vi "ide_comandos.vi"() -> ()   [LabVIEW 2011]
uses:
  <vilib>/addons/System Identification/Model Conversion.llb/SI Convert to Transfer Function Model of CDT.vi
  <vilib>/addons/Control Design/_Utility/Model Viewer.llb/Model Viewer SubVI/cd_Draw Transfer Function Equation (TF).vi
  <vilib>/addons/Control Design/_Time Response Analysis/Time Response.llb/Time Response subVI/cd_Step Response (Transfer Function).vi
  <vilib>/addons/System Identification/NI_SysID.lvlib
  <vilib>/addons/Control Design/_Time Response Analysis/NI_CD_Time Response.lvlib
  <vilib>/addons/Control Design/_Utility/NI_CD_Model Viewer.lvlib
panel:
  out "MODELO ARX TIEMPO DISCRETO":picture
  out "FUNCION DE TRANSF. TIEMPO CONT.":picture
  in  "model type":u16(ring)=1 items=["State-Space", "Transfer Function", "Zero-Pole-Gain"]
  out "RESPUESTA AL ESCALON":cluster{"time":dbl[], dbl[]}[](graph)=[{"time"=[0.0, 0.020293175540355358, 0.040586351080710716, 0.06087952662106608, 0.08117270216142143, 0.10146587770177679, 0.12175905324213215, 0.1420522287824875, 0.16234540432284286, 0.18263857986319823, 0.20293175540355357, 0.22322493094390894, 0.2435181064842643, 0.2638112820246197, 0.284104457564975, 0.30439763310533036, 0.3246908086456857, 0.3449839841860411, 0.36527715972639646, 0.3855703352667518, 0.40586351080710714, 0.4261566863474625, 0.4464498618878179, 0.46674303742817325, 0.4870362129685286, 0.507329388508884, 0.5276225640492394, 0.5479157395895946, 0.56820891512995, 0.5885020906703053, 0.6087952662106607, 0.6290884417510161, 0.6493816172913714, 0.6696747928317268, 0.6899679683720822, 0.7102611439124376, 0.7305543194527929, 0.7508474949931483, 0.7711406705335035, 0.7914338460738589, 0.8117270216142143], [0.0, 0.18042870525480673, 0.32815123498496285, 0.44909621299752056, 0.548117585926744, 0.6291894291559041, 0.6955654404163361, 0.7499095221019031, 0.7944026930256598, 0.8308306203628951, 0.8606552847447804, 0.8850736546744598, 0.9050657250759233, 0.9214338479313019, 0.9348349334831595, 0.9458068143490943, 0.9547898306331434, 0.9621445023202948, 0.9681659982093576, 0.9730959820732661, 0.9771323114748264, 0.9804369784854365, 0.9831426109957054, 0.9853577955383902, 0.9871714352472293, 0.9886563178518591, 0.9898720369049804, 0.9908673834808734, 0.9916823043325279, 0.9923495050951021, 0.9928957628778988, 0.9933430009237824, 0.993709168465894, 0.9940089610933998, 0.9942544105370846, 0.9944553675449554, 0.9946198972273457, 0.9947546027381128, 0.9948648902823868, 0.9949551860865656, 0.9950291140383205]}]
  in  "Filename":path=path "B:/UNI/Control Digital/2013-II/Laboratorios en el MT/7/circuito_rc.sim"
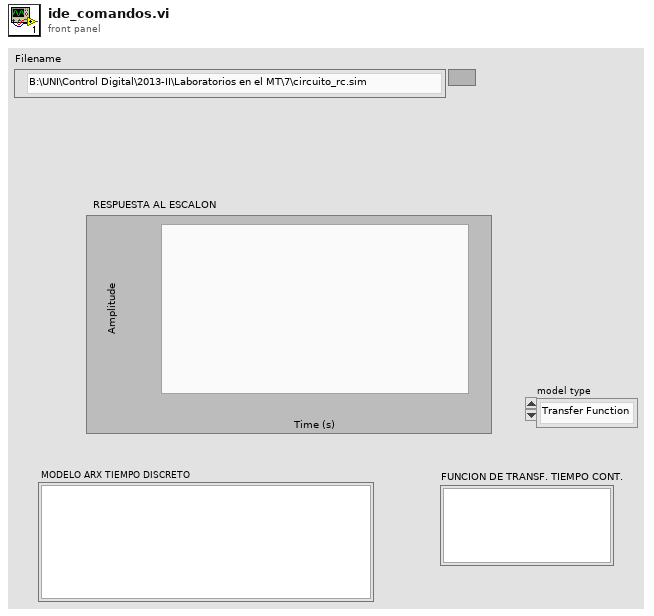
[diagram p1: front panel]
types:
  T1 = typedef "NI_SysID.lvlib/si_generic model.ctl" = cluster{"attributes":cluster{"version":string, "model type":T2, "input names":string[], "output names":string[], "notes":string}, "coefficients":cluster{"A ":dbl[][][], "B":dbl[][][], "F":dbl[][][], "C":dbl[][][], "D":dbl[][][]}, "std deviations":cluster{"A ":dbl[][][], "B":dbl[][][], "F":dbl[][][], "C":dbl[][][], "D":dbl[][][]}, "coefficients covariance":dbl[][][], "noise variance":dbl[][], "fs":dbl, "system info":cluster{"number of inputs":i32, "number of outputs":i32, "A order":i32[][], "B order":i32[][], "F order":i32[][], "C order":i32[][], "D order":i32[][], "Delays":i32[][]}, "kalman gain":dbl[][], "initial state":dbl[], "trans func":cluster{"betas":dbl[], "alphas":dbl[]}[][], "zeros-poles":cluster{"zeros":cdb[], "poles":cdb[], "gain":dbl}[][], "std of trans func":cluster{"betas":dbl[], "alphas":dbl[]}[][], "std of zeros-poles":cluster{"zeros":cdb[], "poles":cdb[], "gain":dbl}[][], "trans func (noise)":cluster{"betas":dbl[], "alphas":dbl[]}[][], "std of trans func (noise)":cluster{"betas":dbl[], "alphas":dbl[]}[][], "zeros-poles (noise)":cluster{"zeros":cdb[], "poles":cdb[], "gain":dbl}[][], "std of zeros-poles (noise)":cluster{"zeros":cdb[], "poles":cdb[], "gain":dbl}[][], "Symbolic State Space Model":cluster{"Symbolic A":string[][], "Symbolic B":string[][], "Symbolic C":string[][], "Symbolic D":string[][], "Symbolic K":string[][], "Symbolic Initial State":string[]}, "delay":dbl[][], "variables":T3, "grey trans func spec":cluster{"orders of TF model":cluster{" num order":i32, "den order":i32}, "# of zeros/poles at origin":cluster{"zeros/poles":u16, "number ":i32}, "delay initial?":bool, "gain initial?":bool}}
  T2 = typedef "NI_SysID.lvlib/SI Model Type.ctl" = u16
  T3 = typedef "NI_SysID.lvlib/si_variables.ctl" = cluster{"name":string, "initial guess":dbl, "upper limit":dbl, "lower limit":dbl, "value":dbl}[]
  T4 = typedef "NI_LinSys_Model Typedefs.lvlib/CD Transfer Function Model (MIMO).ctl" = cluster{"properties":T5, "transfer function(s)":T6[][]}
  T5 = typedef "NI_LinSys_Model Typedefs.lvlib/CD General Elements.ctl" = cluster{"Model name":string, "Input names":string[], "Output names":string[], "Input Delays":dbl[], "Output Delays":dbl[], "Sampling Time":dbl, "Notes":string}
  T6 = typedef "NI_LinSys_Model Typedefs.lvlib/CD Transfer Function Model (SISO).ctl" = cluster{"Numerator":dbl[], "Denominator":dbl[], "delay":dbl}
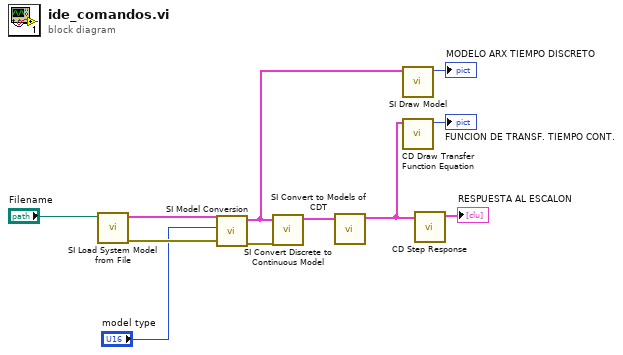
[diagram p0: block diagram]
diagram:
  n1 = call <vilib>:"SI Load System Model from File.vi"("file path"="Filename") -> ("error out"=w9:errorcluster, "system model"=w8:T1)  [unwired: 7 in, 2 out]
  n2 = call <vilib>:"SI Model Conversion.vi"("error in (no error)"=w9, "model type"="model type", "system model in"=w8) -> ("error out"=w11:errorcluster, "system model out"=w7:T1)  [unwired: 7 in]
  n3 = call <vilib>:"SI Convert Discrete to Continuous Model.vi"("error in (no error)"=w11, "system model in"=w7) -> ("system model out"=w6:T1)  [unwired: 8 in, 1 out]
  n4 = call-poly <vilib>:"SI Convert to Models of CDT.vi"("system model"=w6) -> ("transfer function model"=w5:T4)  [unwired: 9 in, 1 out]
  n5 = call <vilib>:"SI Draw Model.vi"("system model"=w7) -> ("model"=→"MODELO ARX TIEMPO DISCRETO":picture)  [unwired: 8 in, 2 out]
  n6 = call-poly <vilib>:"CD Draw Transfer Function Equation.vi"("Transfer Function Model"=w5) -> ("Equation"=→"FUNCION DE TRANSF. TIEMPO CONT.":picture)  [unwired: 8 in, 2 out]
  n7 = call-poly <vilib>:"CD Step Response.vi"("Transfer Function Model"=w5) -> ("Step Response Graph"=→"RESPUESTA AL ESCALON":cluster{"time":dbl[], dbl[]}[])  [unwired: 8 in, 2 out]
